vi "06Foot.vi"() -> ()   [LabVIEW 2015]
uses:
  <vilib>/DAQmx/create/channels.llb/DAQmx Create Channel (DI-Digital Input).vi
  <vilib>/DAQmx/configure/timing.llb/DAQmx Timing (Sample Clock).vi
  <vilib>/Utility/file.llb/Write Delimited Spreadsheet (DBL).vi
panel:
  in  "Tab Control":T1(tab)
  out "ms elapsed":u32
  out "data":u8[](array[numeric])
  out "Array 5":u32[](array[numeric])
  out "Read":dbl[](array[numeric])
  out "Waveform Graph 1":dbl[](graph)
  out "Waveform Graph 2":dbl[](graph)
  out "Waveform Graph 3":dbl[](graph)
  out "Waveform Graph 4":dbl[](graph)
  out "Waveform Graph":dbl[][](graph)
  in  "stop":bool
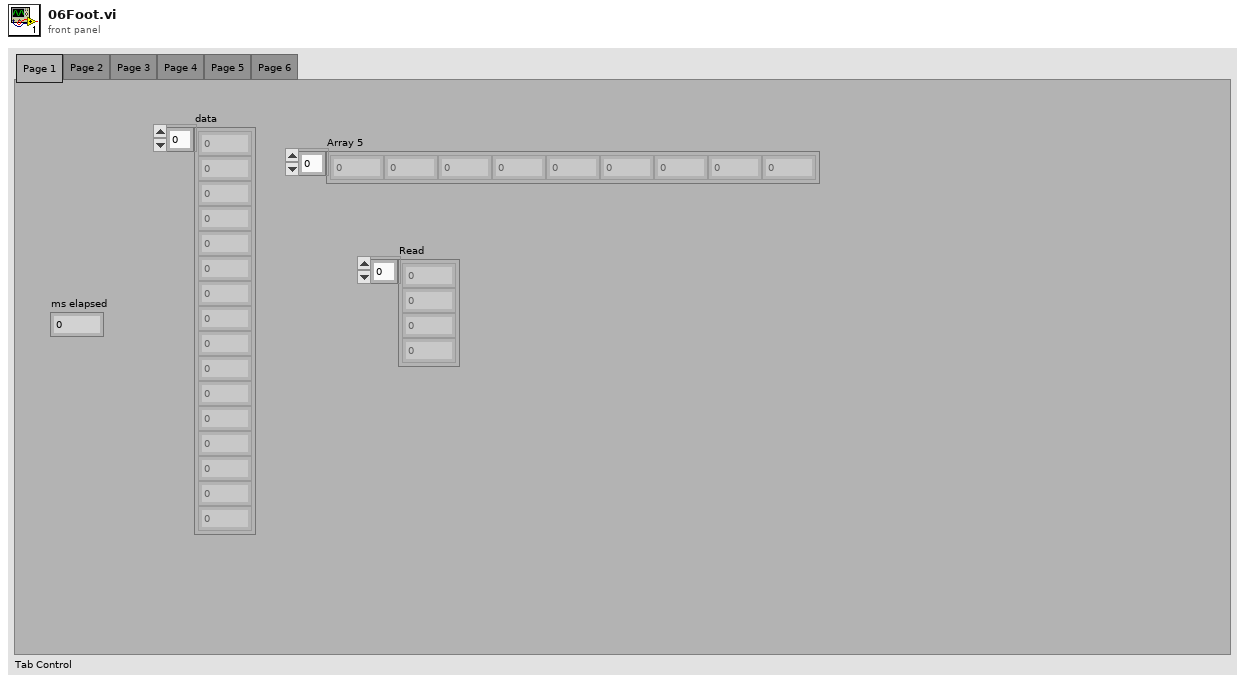
[diagram p1: front panel]
types:
  T1 = enum32{"Page 1", "Page 2", "Page 3", "Page 4", "Page 5", "Page 6"}
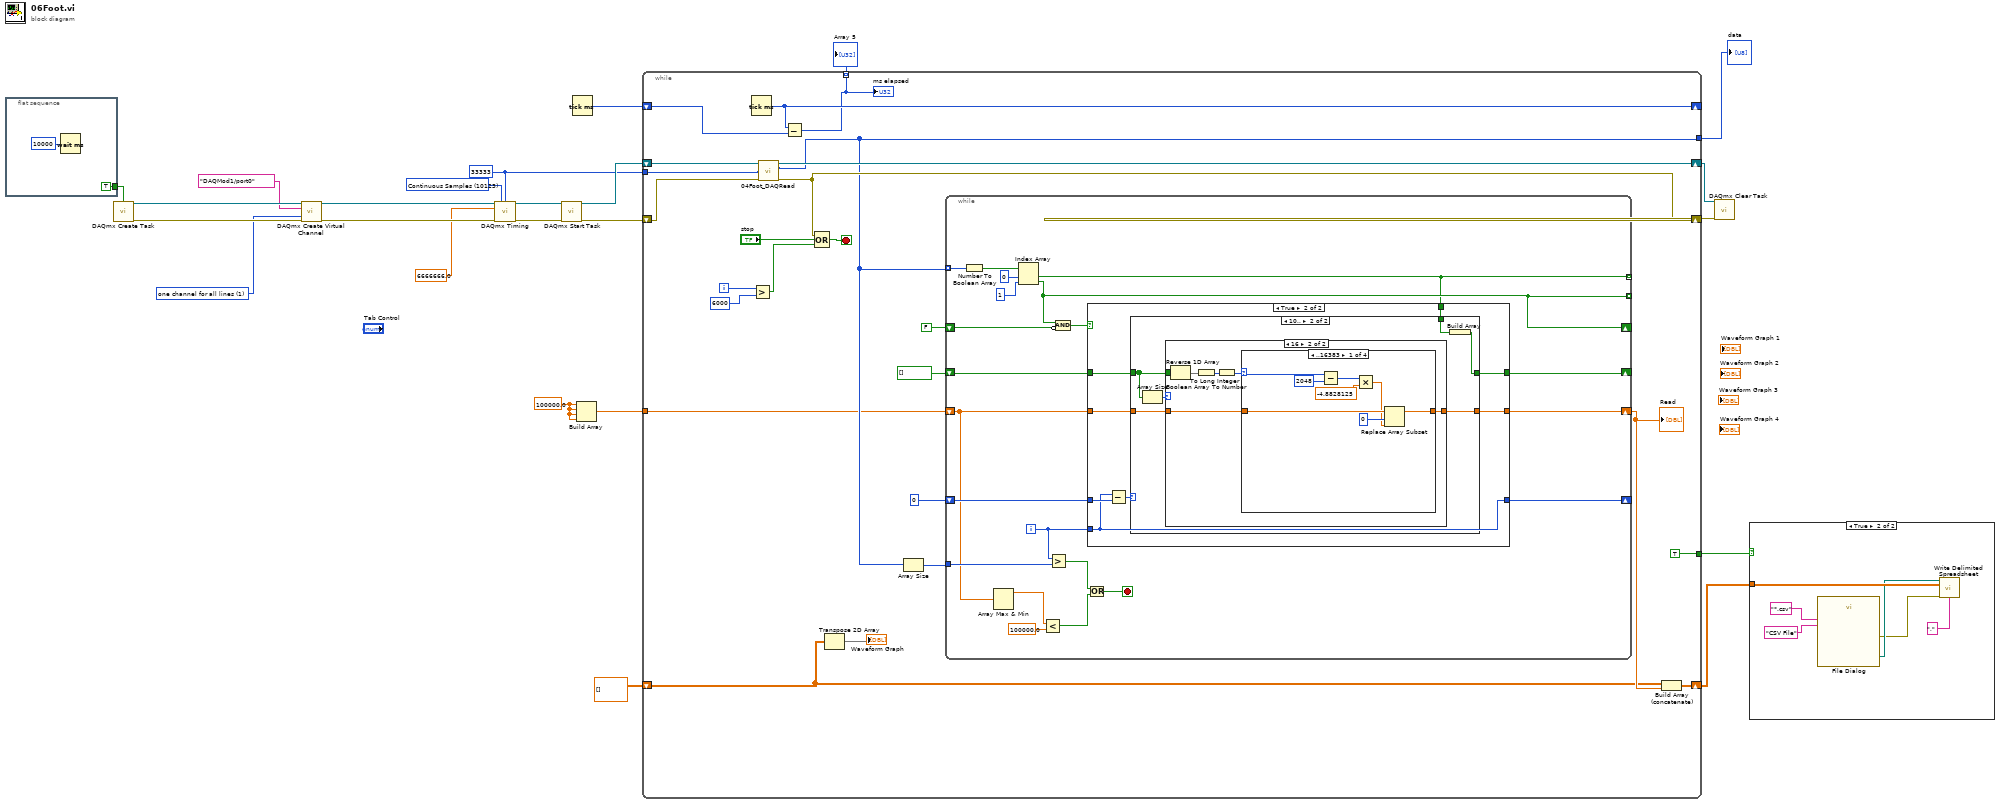
[diagram p0: block diagram]
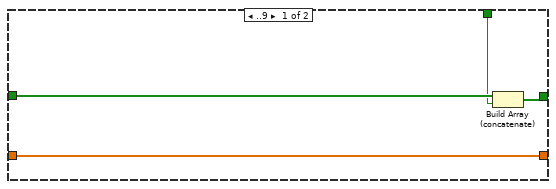
[diagram p4: hidden frame]
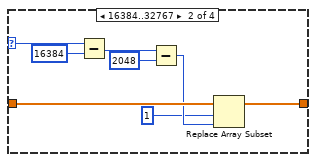
[diagram p6: hidden frame]
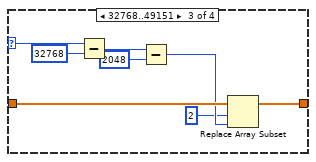
[diagram p7: hidden frame]
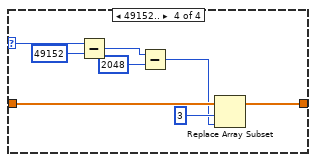
[diagram p8: hidden frame]
diagram:
  w4 = 100000.0 ("element")
  w11 = 33333 ("samples per channel")
  w12 = 10123 items=["Finite Samples"=10178, "Continuous Samples"=10123, "Hardware Timed Single Point"=12522] ("sample mode")
  w14 = 1 items=["one channel for each line", "one channel for all lines"] ("line grouping")
  n1 = flat-sequence {
    tunnel: [TRUE ("auto cleanup")] -> w10
    frame #0 {
      n2 = Wait (ms)(milliseconds to wait=u32 10000) -> ()  [unwired: 1 out]
    }
  }
  n3 = call <vilib>:"DAQmx Create Task.vi"("auto cleanup"=w10) -> ("task out"=w21:refnum<k21>, "error out"=w20:errorcluster)  [unwired: 13 in]
  n4 = call-poly <vilib>:"DAQmx Create Virtual Channel.vi"("task in"=w21, "lines"=tag "DAQMod1/port0", "line grouping"=w14, "error in"=w20) -> ("task out"=w23:refnum<k21>, "error out"=w22:errorcluster)  [unwired: 10 in]
  n5 = call-poly <vilib>:"DAQmx Timing.vi"("task/channels in"=w23, "sample mode"=w12, "samples per channel"=w11, "rate"=6666666.0, "error in"=w22) -> ("task out"=w19:refnum<k21>, "error out"=w18:errorcluster)  [unwired: 9 in]
  n6 = call <vilib>:"DAQmx Start Task.vi"("task/channels in"=w19, "error in"=w18) -> ("task out"=w16:refnum<k21>, "error out"=w17:errorcluster)  [unwired: 12 in]
  n7 = Tick Count (ms)() -> (millisecond timer value=w24:u32)
  n8 = Build Array(w4, w4, w4, w4) -> (w3:dbl[])
  n9 = while {
    shift-right: [w50] -> _
    shift-left: w24 -> [w49]
    shift-right: [w34] -> w8
    shift-left: w17 -> [w35]
    shift-right: [w37] -> w9
    shift-left: w16 -> [w38]
    tunnel: w11 -> [w36]
    tunnel: [w32] -> w7
    tunnel: [w43] -> w6 mode=indexing
    shift-right: [w42] -> w2
    shift-left: dbl[][] [] -> [w28]
    tunnel: w3 -> [w30]
    tunnel: [TRUE] -> w1
    i -> [w41]
    stop <- w48 stop-if-true
    n10 = Tick Count (ms)() -> (millisecond timer value=w50:u32)
    n11 = Greater?(x=w41, y=6000) -> (0:w39:bool)
    n12 = call "04Foot_DAQRead.vi"("task/channels in"=w38, "number of samples per channel"=w36, "error in"=w35) -> ("task out"=w37:refnum<k21>, "data"=w32:u8[], "error out"=w34:errorcluster)  [unwired: 10 in]
    n13 = Subtract(x=w50, y=w49) -> (x-y=w43:u32)
    "ms elapsed" <- w43
    n14 = Compound Arithmetic op=OR(w34, "stop", w39) -> (w48:bool)
    n15 = Transpose 2D Array(2D array=w28) -> (transposed array=→"Waveform Graph":dbl[][])
    n16 = Array Size(array=w32) -> (size(s)=w31:i32)
    n17 = while {
      tunnel: w32 -> [w71] mode=indexing
      tunnel: [w62] -> _ mode=indexing
      tunnel: [w67] -> _ mode=indexing
      shift-right: [w67] -> _
      shift-left: FALSE -> [w66]
      shift-right: [w63] -> _
      shift-left: 0 -> [w64]
      shift-right: [w61] -> _
      shift-left: bool[] [] -> [w60]
      tunnel: w31 -> [w57]
      shift-right: [w59] -> w33
      shift-left: w30 -> [w56]
      i -> [w58]
      stop <- w53 stop-if-true
      n18 = Number To Boolean Array(number=w71) -> (Boolean array=w70:bool[])
      n19 = Array Max & Min(array=w56) -> (max value=w55:dbl)  [unwired: 3 out]
      n20 = Index Array(array=w70, index #1=0 ("index"), index #2=1 ("index")) -> (element #1=w62:bool, element #2=w67:bool)
      n21 = Less?(x=w55, y=100000.0) -> (x < y?=w52:bool)
      n22 = Greater?(x=w58, y=w57) -> (0:w51:bool)
      n23 = Compound Arithmetic op=AND(w67, invert w66) -> (w65:bool)
      n24 = Or(x=w51, y=w52) -> (x .or. y?=w53:bool)
      n25 = case shown="True" w65 {
        tunnel: w58 -> [_ w80]
        tunnel: w64 -> [w74 w82]
        tunnel: [w74 w80] -> w63
        tunnel: w62 -> [_ w79]
        tunnel: [w73 w77] -> w61
        tunnel: w60 -> [w73 w78]
        tunnel: [w72 w75] -> w59
        tunnel: w56 -> [w72 w76]
        frame False {
        }
        frame True {
          n26 = Subtract(x=w80, y=w82) -> (x-y=w81:i32)
          n27 = case shown="10.." w81 {
            tunnel: w79 -> [w85 w91]
            tunnel: w78 -> [w86 w87]
            tunnel: [w84 w92] -> w77
            tunnel: w76 -> [w83 w90]
            tunnel: [w83 w89] -> w75
            frame ..9 {
              n28 = Build Array (concatenate)(w86, w85) -> (w84:bool[])
            }
            frame 10.. {
              n29 = Array Size(array=w87) -> (size(s)=w88:i32)
              n30 = case shown="16" w88 {
                tunnel: w87 -> [_ w99]
                tunnel: w90 -> [w93 w97]
                tunnel: [w93 w96] -> w89
                frame 0, Default {
                }
                frame 16 {
                  n31 = Reverse 1D Array(array=w99) -> (reversed array=w98:bool[])
                  n32 = Boolean Array To Number(Boolean array=w98) -> (number=w95:u32)
                  n33 = To Long Integer(number=w95) -> (32bit integer=w94:i32)
                  n34 = case shown="..16383" w94 {
                    selector: w94 -> [w107 w115 w123 w131]
                    tunnel: w97 -> [w103 w111 w119 w127]
                    tunnel: [w100 w108 w118 w126] -> w96
                    frame ..16383 {
                      n35 = Subtract(x=w107, y=2048) -> (x-y=w105:i32)
                      n36 = Multiply(x=w105, y=-4.8828125) -> (x*y=w101:dbl)
                      n37 = Replace Array Subset(array=w103, new element=w101, index=0) -> (w100:dbl[])
                    }
                    frame 16384..32767 {
                      n38 = Subtract(x=w115, y=16384) -> (x-y=w113:i32)
                      n39 = Subtract(x=w113, y=2048) -> (x-y=w110:i32)
                      n40 = Replace Array Subset(array=w111, new element=w110, index=1) -> (w108:dbl[])
                    }
                    frame 32768..49151 {
                      n41 = Subtract(x=w123, y=32768) -> (x-y=w121:i32)
                      n42 = Subtract(x=w121, y=2048) -> (x-y=w117:i32)
                      n43 = Replace Array Subset(array=w119, new element=w117, index=2) -> (w118:dbl[])
                    }
                    frame 49152.. {
                      n44 = Subtract(x=w131, y=49152) -> (x-y=w129:i32)
                      n45 = Subtract(x=w129, y=2048) -> (x-y=w124:i32)
                      n46 = Replace Array Subset(array=w127, new element=w124, index=3) -> (w126:dbl[])
                    }
                  }
                }
              }
              n47 = Build Array(w91) -> (w92:bool[])
            }
          }
        }
      }
    }
    "Read" <- w33
    n48 = Build Array (concatenate)(w28, w33) -> (w42:dbl[][])
  }
  "data" <- w7
  "Array 5" <- w6
  n49 = call <vilib>:"DAQmx Clear Task.vi"("task in"=w9, "error in"=w8) -> ()  [unwired: 13 in, 1 out]
  n50 = case shown="True" w1 {
    tunnel: w2 -> [_ w136]
    frame False {
    }
    frame True {
      n51 = call "File Dialog"("pattern (all files)"="*.csv", "pattern label"="CSV File") -> ("selected path"=w135:path, "error out"=w134:errorcluster)  [unwired: 10 in, 2 out]
      n52 = call-poly <vilib>:"Write Delimited Spreadsheet.vi"("file path (dialog if empty)"=w135, "2D data"=w136, "error in (no error)"=w134, "delimiter (\\t)"="," ("delimiter (\\t)")) -> ()  [unwired: 10 in, 2 out]
    }
  }
